vi "Main Subpanel.vi"() -> ()   [LabVIEW 2015]
panel:
  in  "stop":bool
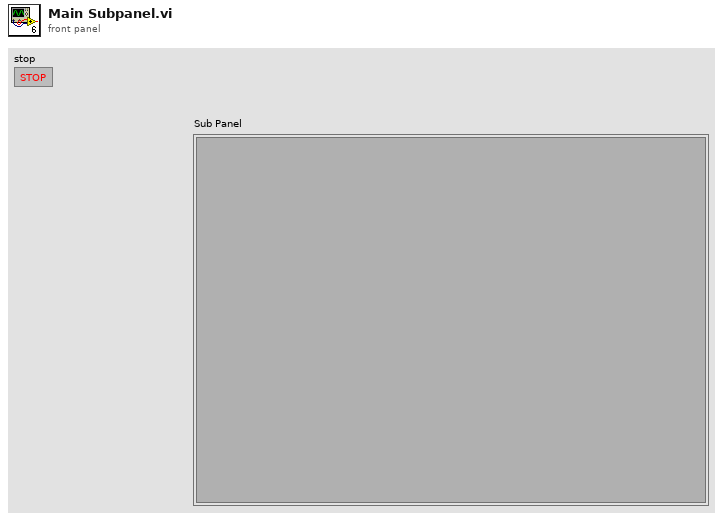
[diagram p1: front panel]
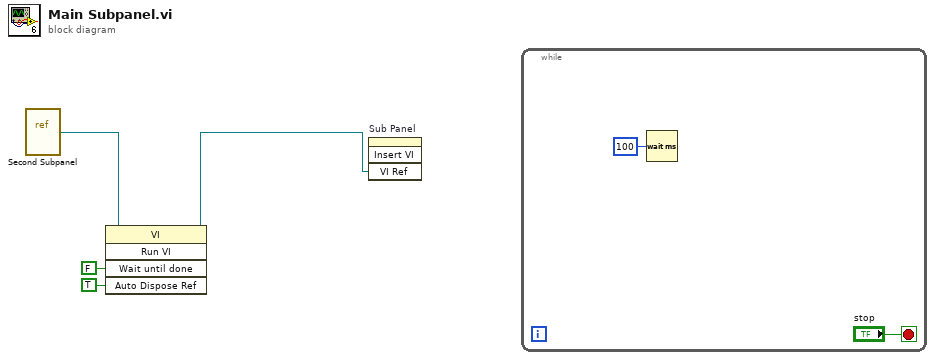
[diagram p0: block diagram]
diagram:
  n1 = vi-ref "Second Subpanel.vi"() -> (w4:refnum<vi>)
  n2 = invoke class="VI" method="Run VI"(reference=w4, "Wait until done"=FALSE ("Wait Until Done"), "Auto Dispose Ref"=TRUE ("Auto Dispose Reference")) -> (reference out=w3:refnum<vi>)  [unwired: 2 in, 4 out]
  n3 = invoke on="Sub Panel" class="SubPnl" method="Insert VI"("VI Ref"=w3) -> ()  [unwired: 3 in, 4 out]
  n4 = while {
    stop <- "stop" stop-if-true
    n5 = Wait (ms)(milliseconds to wait=u32 100) -> ()  [unwired: 1 out]
  }
